vi "5790A_init.vi"(0 "5790A":refnum<visa-resource-name>, 2 "reset (T:yes)":bool, 3 "ID? (T:yes)":bool, 5 "error in":errorcluster) -> (6 "Session Out":refnum<visa-resource-name>, 7 "ID":string, 8 "error out":errorcluster)   [LabVIEW 2020]
doc: "this vi initializes the Datron 4xxx calibrator"
uses:
  <vilib>/Instr/_visa.llb/VISA GPIB Control REN Mode.ctl
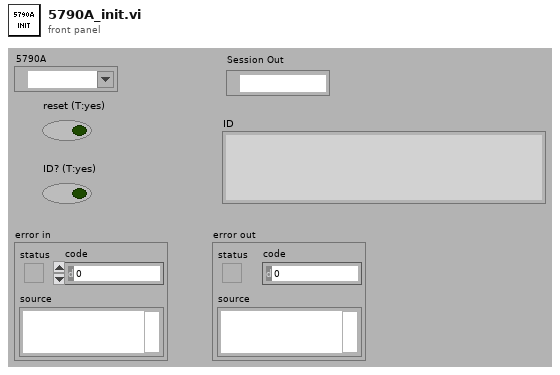
[diagram p1: front panel]
types:
  T1 = typedef "VISA GPIB Control REN Mode.ctl" = u16
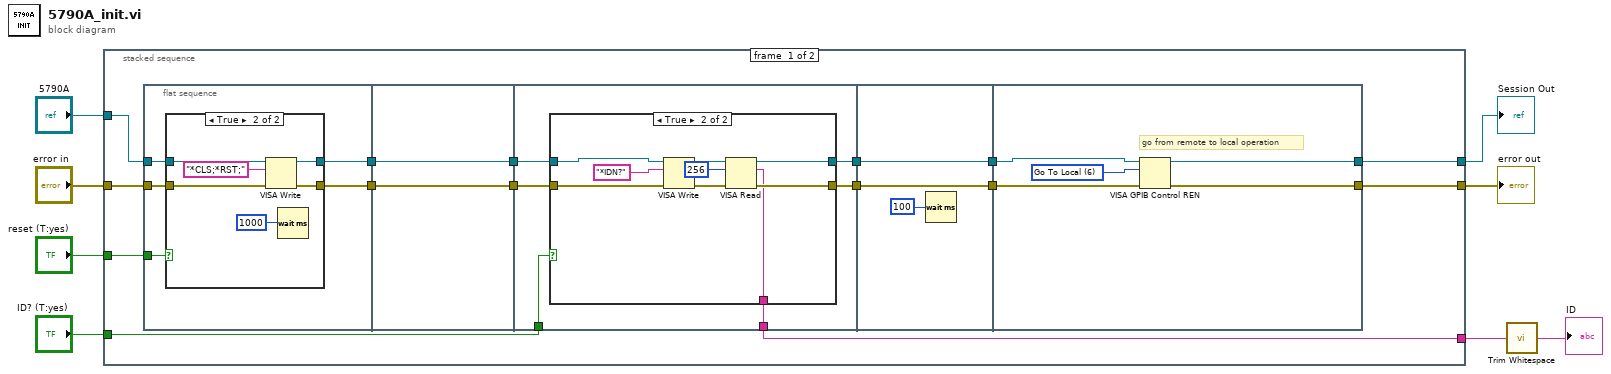
[diagram p0: block diagram]
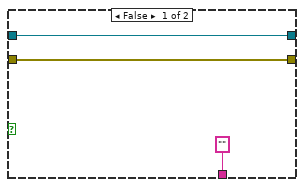
[diagram p3: hidden frame]
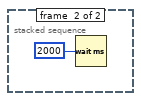
[diagram p4: hidden frame]
diagram:
  n1 = stacked-sequence {
    tunnel: "5790A" -> [w19 _]
    tunnel: [w22 _] -> w7
    tunnel: "error in" -> [w18 _]
    tunnel: [w23 _] -> w5
    tunnel: "reset (T:yes)" -> [w17 _]
    tunnel: "ID? (T:yes)" -> [w10 _]
    tunnel: [w9 _] -> w2
    frame #0 {
      n2 = flat-sequence {
        tunnel: [w24] -> w21
        tunnel: [w25] -> w20
        tunnel: w19 -> [w27]
        tunnel: w18 -> [w26]
        tunnel: w17 -> [w28]
        tunnel: [w38] -> w16
        tunnel: [w37] -> w15
        tunnel: w21 -> [w37]
        tunnel: w20 -> [w38]
        tunnel: w16 -> [w43]
        tunnel: [w41] -> w14
        tunnel: w15 -> [w42]
        tunnel: [w40] -> w12
        tunnel: w10 -> [w44]
        tunnel: [w39] -> w9
        tunnel: w14 -> [w59]
        tunnel: [w59] -> w13
        tunnel: w12 -> [w58]
        tunnel: [w58] -> w11
        tunnel: [w64] -> w22
        tunnel: [w63] -> w23
        tunnel: w13 -> [w61]
        tunnel: w11 -> [w60]
        frame #0 {
          n3 = case shown="True" w28 {
            tunnel: w27 -> [w30 w36]
            tunnel: w26 -> [w29 w35]
            tunnel: [w30 w34] -> w25
            tunnel: [w29 w33] -> w24
            frame False {
            }
            frame True {
              n4 = VISA Write(VISA resource name=w36, write buffer="*CLS;*RST;", error in (no error)=w35) -> (VISA resource name out=w34:refnum<visa-resource-name>, error out=w33:errorcluster)  [unwired: 1 out]
              n5 = Wait (ms)(milliseconds to wait=u32 1000) -> ()  [unwired: 1 out]
            }
          }
        }
        frame #1 {
        }
        frame #2 {
          n6 = case shown="True" w44 {
            tunnel: w43 -> [w47 w56]
            tunnel: w42 -> [w46 w55]
            tunnel: [w47 w50] -> w41
            tunnel: [w46 w52] -> w40
            tunnel: ["" ("read buffer") w48] -> w39
            frame False {
            }
            frame True {
              n7 = VISA Write(VISA resource name=w56, write buffer="*IDN?", error in (no error)=w55) -> (VISA resource name out=w51:refnum<visa-resource-name>, error out=w53:errorcluster)  [unwired: 1 out]
              n8 = VISA Read(VISA resource name=w51, byte count=u32 256, error in (no error)=w53) -> (VISA resource name out=w50:refnum<visa-resource-name>, read buffer=w48:string, error out=w52:errorcluster)  [unwired: 1 out]
            }
          }
        }
        frame #3 {
          n9 = Wait (ms)(milliseconds to wait=u32 100) -> ()  [unwired: 1 out]
        }
        frame #4 {
          w62 = T1 6 items=["Deassert REN", "Assert REN", "Go To Local; Deassert REN ", "Assert REN; Address Device", "Local Lockout (Addressed Devices)", "Local Lockout (This Device)", "Go To Local"] ("Mode")
          # "go from remote to local operation"
          n10 = VISA GPIB Control REN(8:w60, 10:w62, 11:w61) -> (0:w64:errorcluster, 3:w63:refnum<visa-resource-name>)
        }
      }
    }
    frame #1 {
      n11 = Wait (ms)(milliseconds to wait=u32 2000 ("millisecond multiple")) -> ()  [unwired: 1 out]
    }
  }
  "Session Out" <- w5
  "error out" <- w7
  n12 = call <vilib>:"Trim Whitespace.vi"("string"=w2) -> ("trimmed string"=→"ID":string)  [unwired: 1 in]
